vi "Variant to String Value.vi"(8 "error in":errorcluster, 11 "Value":variant) -> (0 "error out":errorcluster, 2 "String":string, 3 "type":T1)   [LabVIEW 2020, in "ConstantErrorsMaker.lvlib"]
uses:
  ConstantErrorsMaker.lvlib
  <vilib>/Utility/Data Type/Type Definitions/Data Type.ctl
  <vilib>/addons/analyzer/_analyzerutils.llb/VIAnUtil Check Type If ErrClust.vi
  <vilib>/Utility/Data Type/NI_Data Type.lvlib
  <userlib>/_OpenG.lib/lvdata/lvdata.llb/openg_variant.lvlib
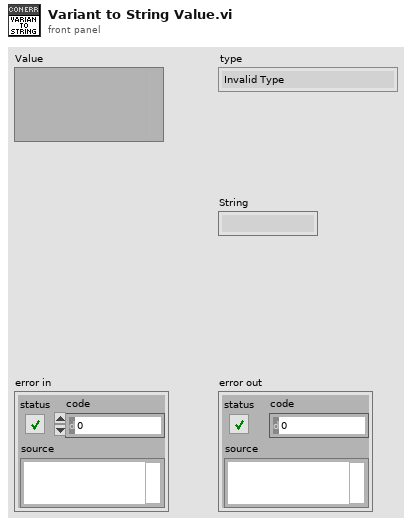
[diagram p1: front panel]
types:
  T1 = typedef "NI_Data Type.lvlib/Data Type.ctl" = enum8{"Invalid Type", "Void", "I8", "I16", "I32", "I64", "U8", "U16", "U32", "U64", "Single Float", "Double Float", "Extended Float", "Single Complex", "Double Complex", "Extended Complex", "Enum U8", "Enum U16", "Enum U32", "Enum U64", "Single Float With Unit", "Double Float With Unit", "Extended Float With Unit", "Single Complex with Unit", "Double Complex with Unit", "Extended Complex with Unit", "Boolean", "String", "Path", "Picture", "Tag", "Array", "Cluster", "Variant", "LV Variant", "Waveform", "Timestamp", "Digital Waveform", "Digital Data", "ExpressData", "Refnum", "External Data", "VI", "Poly VI", "LabVIEW Class Instance", "Fixed Point", "Set Collection", "Map Collection"}
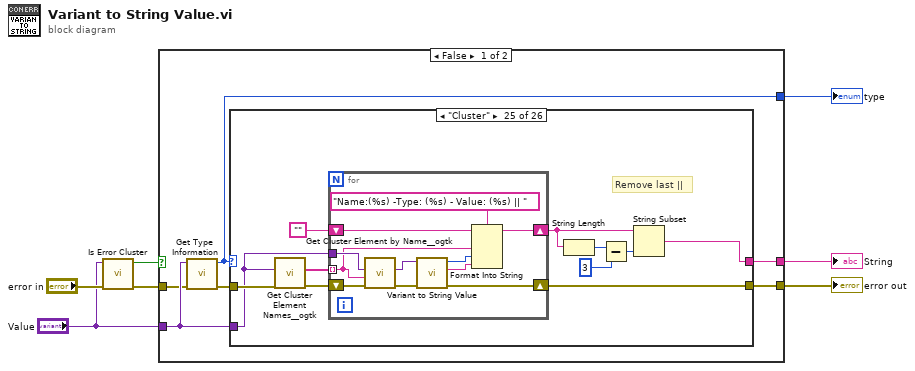
[diagram p0: block diagram]
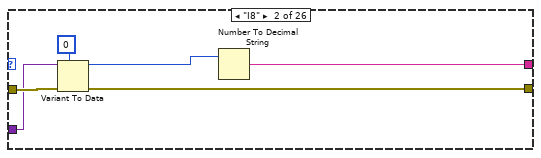
[diagram p3: hidden frame]
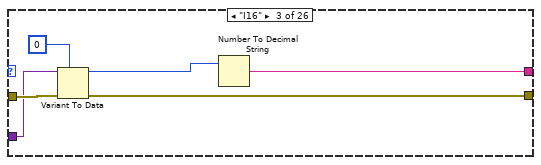
[diagram p4: hidden frame]
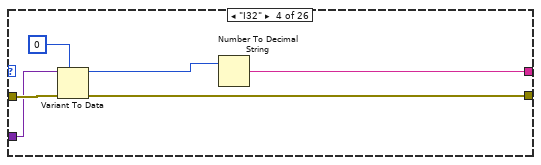
[diagram p5: hidden frame]
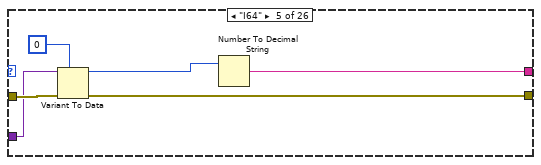
[diagram p6: hidden frame]
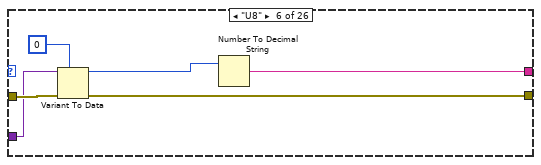
[diagram p7: hidden frame]
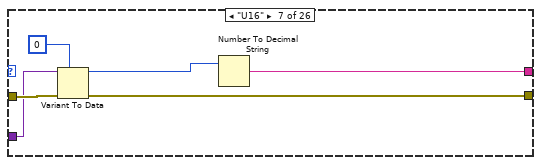
[diagram p8: hidden frame]
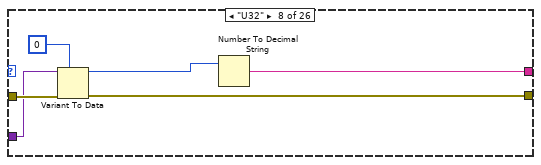
[diagram p9: hidden frame]
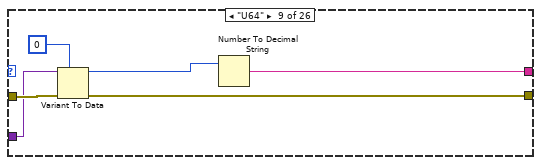
[diagram p10: hidden frame]
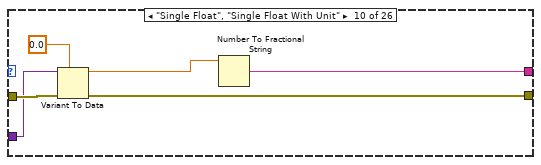
[diagram p11: hidden frame]
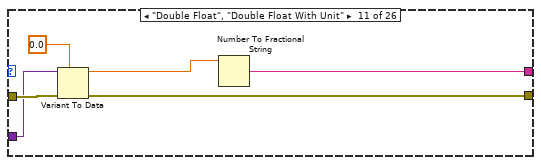
[diagram p12: hidden frame]
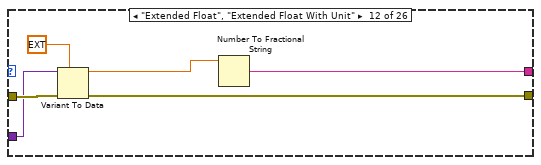
[diagram p13: hidden frame]
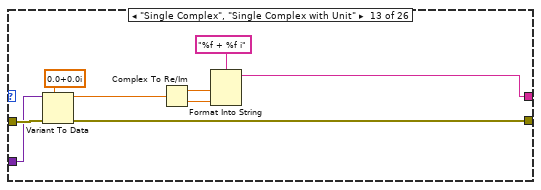
[diagram p14: hidden frame]
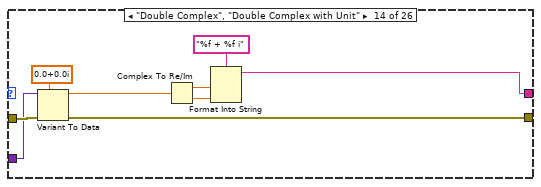
[diagram p15: hidden frame]
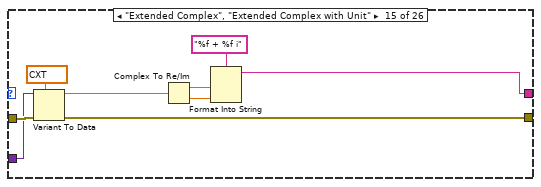
[diagram p16: hidden frame]
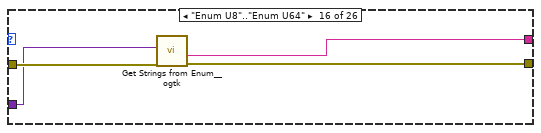
[diagram p17: hidden frame]
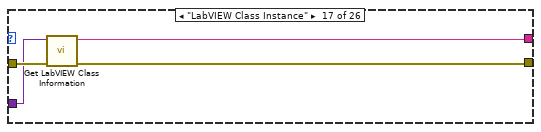
[diagram p18: hidden frame]
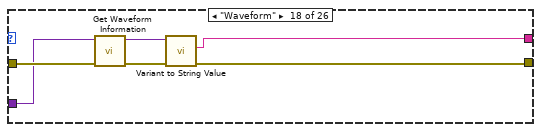
[diagram p19: hidden frame]
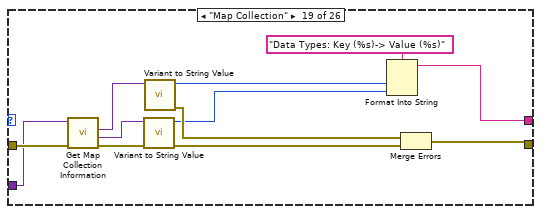
[diagram p20: hidden frame]
diagram:
  n1 = call <vilib>:"Is Error Cluster.vi"("error in (no error)"="error in", "variant"="Value") -> ("error out"=w5:errorcluster, "is error cluster?"=w1:bool)  [unwired: 8 in]
  n2 = case shown="False" w1 {
    tunnel: [w13 w201] -> w7
    tunnel: [w11 Data_Type."Cluster" ("type")] -> w4
    tunnel: [w10 "Error Constant" ("JSON string")] -> w3
    tunnel: w5 -> [w8 w201]
    tunnel: "Value" -> [w9 _]
    frame False {
      n3 = call <vilib>:"Get Type Information.vi"("error in (no error)"=w8, "variant"=w9) -> ("error out"=w12:errorcluster, "type"=w11:T1)  [unwired: 5 in, 3 out]
      n4 = case shown="\"Cluster\"" w11 {
        tunnel: [w14 w19 w25 w31 w37 w43 w49 w55 w61 w67 w73 w79 w88 w97 w106 w110 w114 w119 w130 w139 w146 w151 w157 w165 w177 w197] -> w13
        tunnel: w12 -> [w14 w20 w26 w32 w38 w44 w50 w56 w62 w68 w74 w80 w89 w98 w107 w111 w115 w121 w133 w141 w147 w152 w158 w167 w178 w198]
        tunnel: w9 -> [_ w18 w24 w30 w36 w42 w48 w54 w60 w66 w72 w78 w87 w96 w105 w109 w113 w118 w128 w138 w145 w150 w156 w164 w173 w196]
        tunnel: [_ w15 w21 w27 w33 w39 w45 w51 w57 w63 w69 w75 w84 w93 w102 w108 w112 w116 w123 w135 w142 w148 w153 w160 w172 w192] -> w10
        frame Default {
        }
        frame "I8" {
          n5 = Variant To Data(error in=w20, type=i8 0, Variant=w18) -> (data=w16:i8, error out=w19:errorcluster)
          n6 = Number To Decimal String(number=w16) -> (decimal integer string=w15:string)  [unwired: 1 in]
        }
        frame "I16" {
          n7 = Variant To Data(error in=w26, type=i16 0, Variant=w24) -> (data=w22:i16, error out=w25:errorcluster)
          n8 = Number To Decimal String(number=w22) -> (decimal integer string=w21:string)  [unwired: 1 in]
        }
        frame "I32" {
          n9 = Variant To Data(error in=w32, type=0, Variant=w30) -> (data=w28:i32, error out=w31:errorcluster)
          n10 = Number To Decimal String(number=w28) -> (decimal integer string=w27:string)  [unwired: 1 in]
        }
        frame "I64" {
          n11 = Variant To Data(error in=w38, type=i64 0, Variant=w36) -> (data=w34:i64, error out=w37:errorcluster)
          n12 = Number To Decimal String(number=w34) -> (decimal integer string=w33:string)  [unwired: 1 in]
        }
        frame "U8" {
          n13 = Variant To Data(error in=w44, type=u8 0, Variant=w42) -> (data=w40:u8, error out=w43:errorcluster)
          n14 = Number To Decimal String(number=w40) -> (decimal integer string=w39:string)  [unwired: 1 in]
        }
        frame "U16" {
          n15 = Variant To Data(error in=w50, type=u16 0, Variant=w48) -> (data=w46:u16, error out=w49:errorcluster)
          n16 = Number To Decimal String(number=w46) -> (decimal integer string=w45:string)  [unwired: 1 in]
        }
        frame "U32" {
          n17 = Variant To Data(error in=w56, type=u32 0, Variant=w54) -> (data=w52:u32, error out=w55:errorcluster)
          n18 = Number To Decimal String(number=w52) -> (decimal integer string=w51:string)  [unwired: 1 in]
        }
        frame "U64" {
          n19 = Variant To Data(error in=w62, type=u64 0, Variant=w60) -> (data=w58:u64, error out=w61:errorcluster)
          n20 = Number To Decimal String(number=w58) -> (decimal integer string=w57:string)  [unwired: 1 in]
        }
        frame "Single Float", "Single Float With Unit" {
          n21 = Variant To Data(error in=w68, type=sgl 0.0, Variant=w66) -> (data=w64:sgl, error out=w67:errorcluster)
          n22 = Number To Fractional String(number=w64) -> (F-format string=w63:string)  [unwired: 3 in]
        }
        frame "Double Float", "Double Float With Unit" {
          n23 = Variant To Data(error in=w74, type=0.0, Variant=w72) -> (data=w70:dbl, error out=w73:errorcluster)
          n24 = Number To Fractional String(number=w70) -> (F-format string=w69:string)  [unwired: 3 in]
        }
        frame "Extended Float", "Extended Float With Unit" {
          n25 = Variant To Data(error in=w80, type=ext 0.0, Variant=w78) -> (data=w76:ext, error out=w79:errorcluster)
          n26 = Number To Fractional String(number=w76) -> (F-format string=w75:string)  [unwired: 3 in]
        }
        frame "Single Complex", "Single Complex with Unit" {
          n27 = Variant To Data(error in=w89, type=csg 0.0+0.0i, Variant=w87) -> (data=w85:csg, error out=w88:errorcluster)
          n28 = Complex To Re/Im(x + iy=w85) -> (x=w83:sgl, y=w82:sgl)
          n29 = Format Into String(format string="%f + %f i", w83, w82) -> (resulting string=w84:string)  [unwired: 2 in, 1 out]
        }
        frame "Double Complex", "Double Complex with Unit" {
          n30 = Variant To Data(error in=w98, type=cdb 0.0+0.0i, Variant=w96) -> (data=w94:cdb, error out=w97:errorcluster)
          n31 = Complex To Re/Im(x + iy=w94) -> (x=w92:dbl, y=w91:dbl)
          n32 = Format Into String(format string="%f + %f i", w92, w91) -> (resulting string=w93:string)  [unwired: 2 in, 1 out]
        }
        frame "Extended Complex", "Extended Complex with Unit" {
          n33 = Variant To Data(error in=w107, type=cxt 0.0+0.0i, Variant=w105) -> (data=w103:cxt, error out=w106:errorcluster)
          n34 = Complex To Re/Im(x + iy=w103) -> (x=w101:ext, y=w100:ext)
          n35 = Format Into String(format string="%f + %f i", w101, w100) -> (resulting string=w102:string)  [unwired: 2 in, 1 out]
        }
        frame "Enum U8".."Enum U64" {
          n36 = call <userlib>:"Get Strings from Enum__ogtk.vi"("error in (no error)"=w111, "Enum"=w109) -> ("error out"=w110:errorcluster, "String Value"=w108:string)  [unwired: 6 in, 2 out]
        }
        frame "LabVIEW Class Instance" {
          n37 = call <vilib>:"Get LabVIEW Class Information.vi"("error in (no error)"=w115, "variant"=w113) -> ("error out"=w114:errorcluster, "LabVIEW class file name"=w112:string)  [unwired: 7 in, 1 out]
        }
        frame "Waveform" {
          n38 = call <vilib>:"Get Waveform Information.vi"("error in (no error)"=w121, "variant"=w118) -> ("error out"=w120:errorcluster, "Y array type"=w117:variant)  [unwired: 8 in]
          n39 = call "Variant to String Value.vi"("error in"=w120, "Value"=w117) -> ("error out"=w119:errorcluster, "String"=w116:string)  [unwired: 7 in, 1 out]
        }
        frame "Map Collection" {
          n40 = call <vilib>:"Get Map Collection Information.vi"("error in (no error)"=w133, "variant"=w128) -> ("error out"=w132:errorcluster, "value data type"=w126:variant, "key data type"=w127:variant)  [unwired: 7 in]
          n41 = call "Variant to String Value.vi"("error in"=w132, "Value"=w126) -> ("error out"=w131:errorcluster, "type"=w124:T1)  [unwired: 7 in, 1 out]
          n42 = call "Variant to String Value.vi"("Value"=w127) -> ("error out"=w129:errorcluster, "type"=w125:T1)  [unwired: 8 in, 1 out]
          n43 = Format Into String(format string="Data Types: Key (%s)-> Value (%s)", w125, w124) -> (resulting string=w123:string)  [unwired: 2 in, 1 out]
          n44 = Merge Errors(w129, w131) -> (w130:errorcluster)
        }
        frame "Set Collection" {
          n45 = call <vilib>:"Get Set Collection Information.vi"("error in (no error)"=w141, "variant"=w138) -> ("error out"=w140:errorcluster, "element data type"=w137:variant)  [unwired: 8 in]
          n46 = call "Variant to String Value.vi"("error in"=w140, "Value"=w137) -> ("error out"=w139:errorcluster, "type"=w136:T1)  [unwired: 7 in, 1 out]
          n47 = Format Into String(format string="Data type: (%s)", w136) -> (resulting string=w135:string)  [unwired: 2 in, 1 out]
        }
        frame "Boolean" {
          n48 = Variant To Data(error in=w147, type=TRUE, Variant=w145) -> (data=w143:bool, error out=w146:errorcluster)
          n49 = Format Into String(w143) -> (resulting string=w142:string)  [unwired: 3 in, 1 out]
        }
        frame "String", "Refnum" {
          n50 = Variant To Data(error in=w152, type="", Variant=w150) -> (data=w148:string, error out=w151:errorcluster)
        }
        frame "Path" {
          n51 = Variant To Data(error in=w158, type=path "", Variant=w156) -> (data=w154:path, error out=w157:errorcluster)
          n52 = Path To String(path=w154) -> (string=w153:string)
        }
        frame "Array" {
          n53 = call <vilib>:"Get Array Information.vi"("error in (no error)"=w167, "variant"=w164) -> ("error out"=w166:errorcluster, "array element data type"=w163:variant, "number of dimensions"=w162:i32)  [unwired: 6 in, 1 out]
          n54 = call <vilib>:"Get Type Information.vi"("error in (no error)"=w166, "variant"=w163) -> ("error out"=w165:errorcluster, "type"=w161:T1)  [unwired: 5 in, 3 out]
          n55 = Format Into String(format string="# Dimentions: (%d) - Data Type: (%s)", w162, w161) -> (resulting string=w160:string)  [unwired: 2 in, 1 out]
        }
        frame "Cluster" {
          # "Remove last ||"
          n56 = call <userlib>:"Get Cluster Element Names__ogtk.vi"("error in (no error)"=w178, "Cluster"=w173) -> ("error out"=w176:errorcluster, "Element Names"=w174:string[])  [unwired: 8 in]
          n57 = for {
            tunnel: w173 -> [w186]
            tunnel: w174 -> [w182] mode=indexing
            shift-right: [w184] -> w170
            shift-left: "" -> [w183]
            shift-right: [w187] -> w177
            shift-left: w176 -> [w189]
            n58 = call <userlib>:"Get Cluster Element by Name__ogtk.vi"("error in (no error)"=w189, "Element Name"=w182, "Cluster"=w186) -> ("error out"=w188:errorcluster, "VElement"=w185:variant)  [unwired: 6 in, 1 out]
            n59 = call "Variant to String Value.vi"("error in"=w188, "Value"=w185) -> ("error out"=w187:errorcluster, "String"=w180:string, "type"=w181:T1)  [unwired: 7 in]
            n60 = Format Into String(format string="Name:(%s) -Type: (%s) - Value: (%s) || ", initial string=w183, w182, w181, w180) -> (resulting string=w184:string)  [unwired: 1 in, 1 out]
          }
          n61 = String Length(string=w170) -> (length=w171:i32)
          n62 = Subtract(x=w171, y=3) -> (x-y=w169:i32)
          n63 = String Subset(string=w170, length (rest)=w169) -> (substring=w172:string)  [unwired: 1 in]
        }
        frame "Timestamp" {
          n64 = Variant To Data(error in=w198, type=timestamp(0 s since 1904-01-01), Variant=w196) -> (data=w194:timestamp, error out=w197:errorcluster)
          n65 = Get Date/Time String(seconds (now)=w194) -> (date string=w193:string, time string=w191:string)  [unwired: 2 in]
          n66 = call <vilib>:"Space Constant.vi"() -> ("String"=w190:string)
          n67 = Concatenate Strings(w193, w190, w191) -> (w192:string)
        }
      }
    }
    frame True {
      # "Variant is an Error Cluster"
    }
  }
  "type" <- w4
  "String" <- w3
  "error out" <- w7
